vi "Datasheet Yield Retrieve Channel Results.vi"(8 "error in (no error)":errorcluster, 9 "Test Parameters":T3, 10 "Grouped Results":cluster{"Result Group":T2[]}[](array[cluster])) -> (0 "error out":errorcluster, 2 "Array":T1[](array[typedef]))   [LabVIEW 2011]
uses:
  Datasheet Analysis Parameters.ctl
  www/cgi-bin/_cgi-lib/TDM_INDEX Record.ctl
  CGI Yield Results.ctl
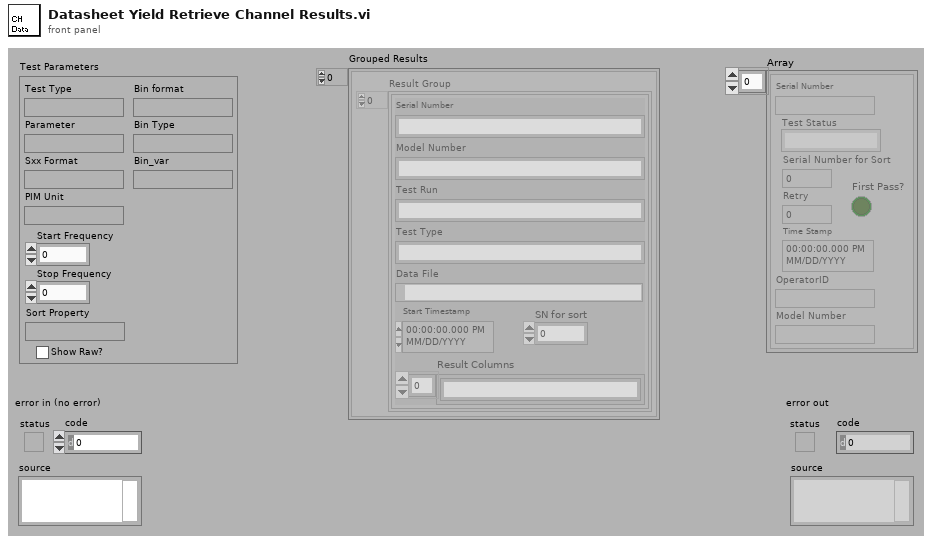
[diagram p1: front panel]
types:
  T1 = typedef "CGI Yield Results.ctl" = cluster{"Model Number":string, "Serial Number for Sort":i32, "Serial Number":string, "Test Status":string, "Time Stamp":timestamp, "OperatorID":string, "Retry":i32, "First Pass?":bool}
  T2 = typedef "TDM_INDEX Record.ctl" = cluster{"Model Number":string, "SN for sort":i32, "Test Type":string, "Test Run":string, "Serial Number":string, "Start Timestamp":timestamp, "Data File":path, "Result Columns":string[]}
  T3 = typedef "Datasheet Analysis Parameters.ctl" = cluster{"Test Type":string, "Parameter":string, "Sxx Format":string, "PIM Unit":string, "Start Frequency":dbl, "Stop Frequency":dbl, "Sort Property":string, "Show Raw?":bool, "Bin format":string, "Bin Type":string, "Bin_var":string}
  T4 = typedef "Connection Refnum.ctl" = cluster{"Environment Handle":i32, "Connection Handle":i32}
  T5 = typedef "Field Record.ctl" = cluster{"ixField":i32, "iSequenceOrder":i32, "sxFieldId":string, "sxSequenceId":string, "sDisplayName":string, "sValue":string, "sUnits":string, "nDataType":T6, "nNextItem":T7, "fSystem":bool, "fSystemValue":bool, "fRequired":bool, "fSetAtTest":bool, "fTestField":bool, "fDeleted":bool, "fIndexed":bool, "fFreeList":bool}
  T6 = typedef "Field DataTypes.ctl" = enum32{"text", "numeric", "list", "timestamp", "boolean"}
  T7 = typedef "Field NextItem.ctl" = enum32{"Reset", "Retain", "Auto-Increment"}
  T8 = typedef "TDMS Model Number.ctl" = cluster{"Model Number":string, "Serial Number Tree Data":T9[]}
  T9 = typedef "TDMS Serial Number.ctl" = cluster{"Serial Number":string, "TDM Files":T10[]}
  T10 = typedef "TDMS File.ctl" = cluster{"File Path":path, "Run Data":T11[], "Serial Number":string, "Model Number":string, "Test Type":string}
  T11 = typedef "TDMS Run.ctl" = cluster{"Channel Data":T12[], "Custom Fields":T5[], "Run ID":string}
  T12 = typedef "TDMS Channel (Sxx).ctl" = cluster{"Channel Name":string, "Waveform":dbl[], "Unit":string, "List value":string}
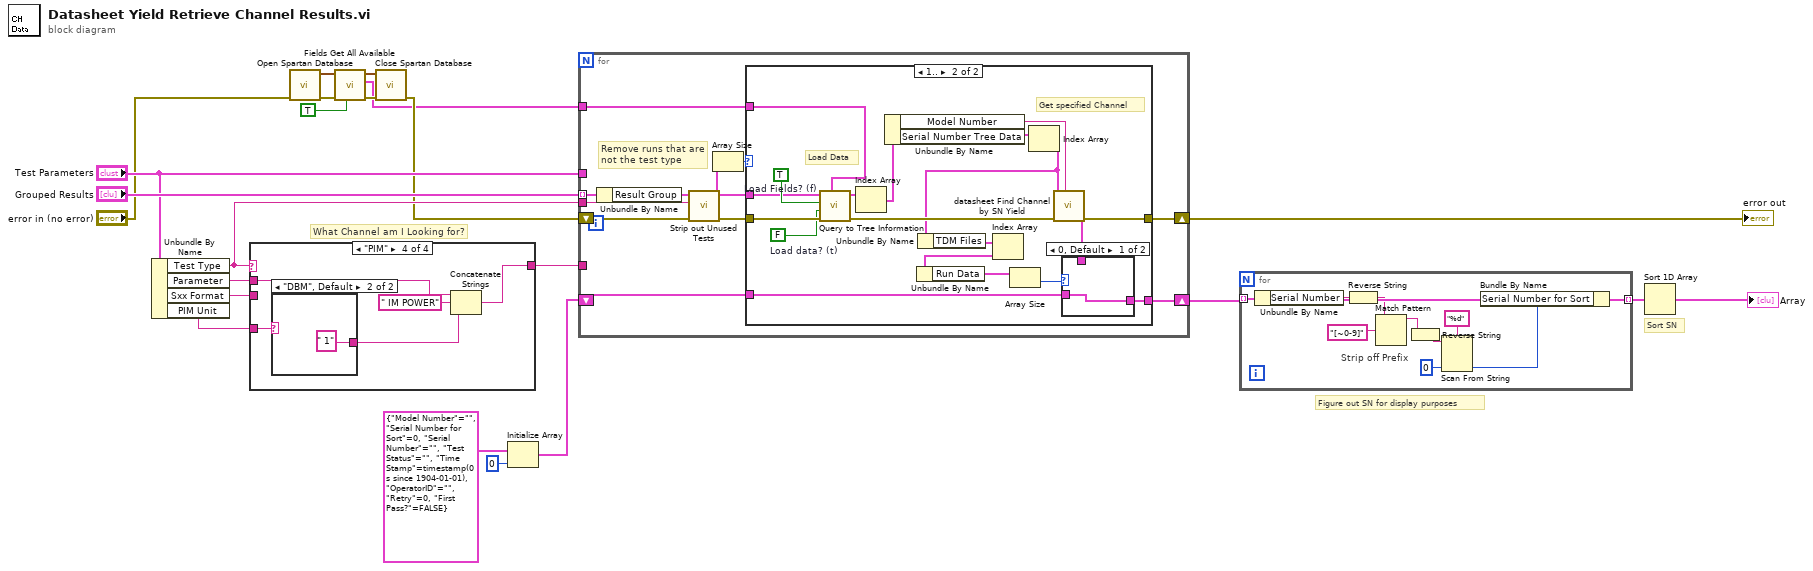
[diagram p0: block diagram]
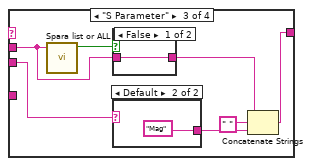
[diagram p4: hidden frame]
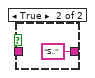
[diagram p5: hidden frame]
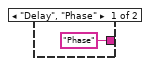
[diagram p6: hidden frame]
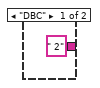
[diagram p7: hidden frame]
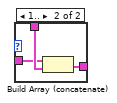
[diagram p9: hidden frame]
diagram:
  # "Sort SN"
  # "Figure out SN for display purposes"
  # "What Channel am I Looking for?"
  n1 = Unbundle By Name("Test Parameters") -> ("Test Type"=w16:string, "Parameter"=w20:string, "Sxx Format"=w19:string, "PIM Unit"=w14:string)
  n2 = case shown="\"PIM\"" w16 {
    tunnel: w20 -> [w23 w24 w25 w39]
    tunnel: w19 -> [_ _ w31 _]
    tunnel: [w23 w24 w29 w40] -> w17
    tunnel: w14 -> [_ _ _ w37]
    frame "Prompted Inputs", Default {
      # "For example find Weight in a\nPrompted Inputs tdm File"
    }
    frame "DC Attenuation" {
      # "For example find ATTN in a\nDC Attenuation  tdm File"
    }
    frame "S Parameter" {
      n3 = call "Spara list or ALL.vi"("S## Type"=w25) -> ("S## List or All?"=w26:bool)  [unwired: 10 out]
      n4 = case shown="False" w26 {
        tunnel: [w32 "S.." ("Property Name")] -> w27
        tunnel: w25 -> [w32 _]
        frame False {
        }
        frame True {
        }
      }
      n5 = case shown="Default" w31 {
        tunnel: ["Phase" ("Property Name") "Mag" ("Property Name")] -> w28
        frame "Delay", "Phase" {
        }
        frame Default {
        }
      }
      n6 = Concatenate Strings(w27, " " ("Property Name"), w28) -> (w29:string)
    }
    frame "PIM" {
      n7 = case shown="\"DBM\", Default" w37 {
        tunnel: [" 2" ("string") " 1" ("string")] -> w36
        frame "DBC" {
        }
        frame "DBM", Default {
        }
      }
      n8 = Concatenate Strings(w39, " IM POWER" ("string"), w36) -> (w40:string)
    }
  }
  n9 = call "Open Spartan Database.vi"("error in (no error)"="error in (no error)") -> ("error out"=w4:errorcluster, "Connection Refnum"=w5:T4)  [unwired: 9 in]
  n10 = call "Fields Get All Available.vi"("Combine All? (f)"=TRUE, "error in (no error)"=w4, "Connection Refnum"=w5) -> ("error out"=w7:errorcluster, "System or ALL Combined Fields"=w1:T5[], "Connection Refnum"=w8:T4)  [unwired: 3 in, 3 out]
  n11 = call "Close Spartan Database.vi"("error in (no error)"=w7, "Connection Refnum"=w8) -> ("error out"=w2:errorcluster)  [unwired: 9 in]
  n12 = Initialize Array(T1 {"Model Number"="", "Serial Number for Sort"=0, "Serial Number"="", "Test Status"="", "Time Stamp"=timestamp(0 s since 1904-01-01), "OperatorID"="", "Retry"=0, "First Pass?"=FALSE} ("Sample Results"), 0 ("dimension size")) -> (w10:T1[])
  n13 = for {
    tunnel: "Test Parameters" -> [_]
    shift-right: [w47] -> w12
    shift-left: w10 -> [w46]
    shift-right: [w49] -> w22
    shift-left: w2 -> [w52]
    tunnel: "Grouped Results" -> [w53] mode=indexing
    tunnel: w17 -> [_]
    tunnel: w16 -> [w48]
    tunnel: w1 -> [w43]
    # "Remove runs that are\nnot the test type"
    n14 = Unbundle By Name(w53) -> ("Result Group"=w50:T2[])
    n15 = call "Strip out Unused Tests.vi"("error in (no error)"=w52, "Test to remain"=w48, "runs"=w50) -> ("error out"=w51:errorcluster, "runs"=w45:T2[])  [unwired: 7 out]
    n16 = Array Size(array=w45) -> (size(s)=w44:i32)
    n17 = case shown="1.." w44 {
      tunnel: w51 -> [w55 w72]
      tunnel: w45 -> [_ w71]
      tunnel: [w55 w67] -> w49
      tunnel: [w54 w64] -> w47
      tunnel: w46 -> [w54 w63]
      tunnel: w43 -> [_ w56]
      frame 0, Default {
      }
      frame 1.. {
        w57 = FALSE  # Load data? (t)
        w73 = TRUE  # Load Fields? (f)
        # "Get specified Channel"
        # "Load Data"
        n18 = call "Query to Tree Information.vi"("System or ALL Combined Fields"=w56, "error in (no error)"=w72, "Load data? (t)"=w57, "Load Fields? (f)"=w73, "Run Array"=w71) -> ("error out"=w68:errorcluster, "Data Tree"=w74:T8[])  [unwired: 5 out]
        n19 = Index Array(array=w74) -> (element=w70:T8)  [unwired: 1 in]
        n20 = Unbundle By Name(w70) -> ("Model Number"=w66:string, "Serial Number Tree Data"=w69:T9[])
        n21 = Index Array(array=w69) -> (element=w62:T9)  [unwired: 1 in]
        n22 = Unbundle By Name(w62) -> ("TDM Files"=w60:T10[])
        n23 = Index Array(array=w60) -> (element=w59:T10)  [unwired: 1 in]
        n24 = Unbundle By Name(w59) -> ("Run Data"=w58:T11[])
        n25 = Array Size(array=w58) -> (size(s)=w61:i32)
        n26 = call "datasheet Find Channel by SN Yield.vi"("Model Number"=w66, "error in (no error)"=w68, "Data"=w62) -> ("error out"=w67:errorcluster, "Sample Results"=w65:T1)  [unwired: 1 in, 6 out]
        n27 = case shown="0, Default" w61 {
          tunnel: w65 -> [_ w78]
          tunnel: [w75 w77] -> w64
          tunnel: w63 -> [w75 w76]
          frame 0, Default {
          }
          frame 1.. {
            n28 = Build Array (concatenate)(w76, w78) -> (w77:T1[])
          }
        }
      }
    }
  }
  "error out" <- w22
  n29 = for {
    tunnel: w12 -> [w87] mode=indexing
    tunnel: [w84] -> w15 mode=indexing
    # "Strip off Prefix"
    n30 = Unbundle By Name(w87) -> ("Serial Number"=w82:string)
    n31 = Reverse String(1:w82) -> (0:w81:string)
    n32 = Match Pattern(string=w81, regular expression="[~0-9]" ("format string")) -> (before substring=w79:string)  [unwired: 4 out]
    n33 = Reverse String(1:w79) -> (0:w80:string)
    n34 = Scan From String(format string="%d", input string=w80, default 1=0 ("default value 1")) -> (output 1=w85:i32)  [unwired: 2 in, 3 out]
    n35 = Bundle By Name(cluster=w87, "Serial Number for Sort"=w85) -> (w84:T1)
  }
  n36 = Sort 1D Array(array=w15) -> (sorted array=→"Array":T1[])
